vi "Просмотр графиков2.vi"(7 "tdm":string) -> ()   [LabVIEW 2011]
panel:
  out "т1 2":waveform(dbl)[](graph)
  out "т1":waveform(dbl)[](graph)
  in  "Закрыть окно":bool
  in  "Сохранить":bool
  # "С1"
  # "С2"
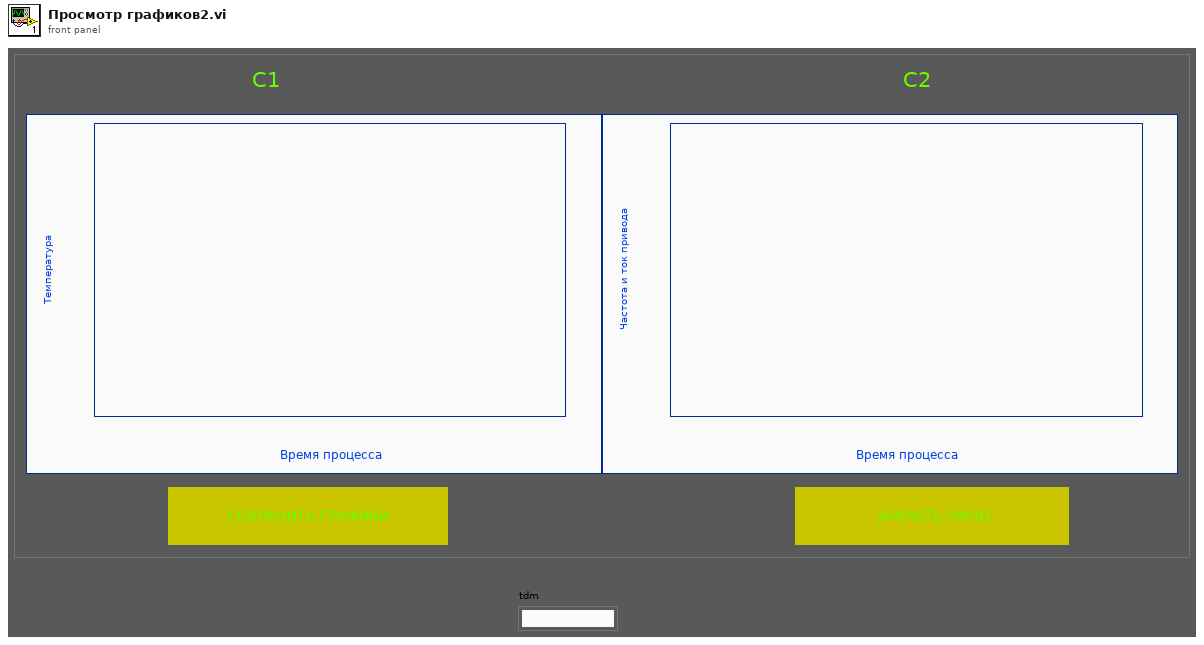
[diagram p1: front panel]
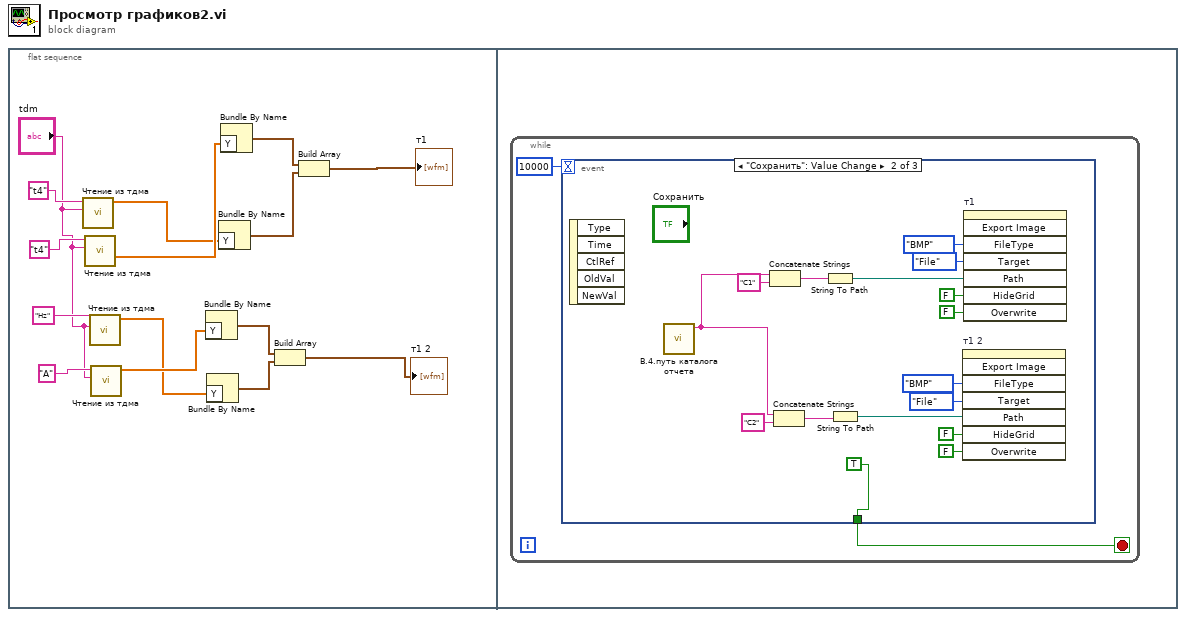
[diagram p0: block diagram]
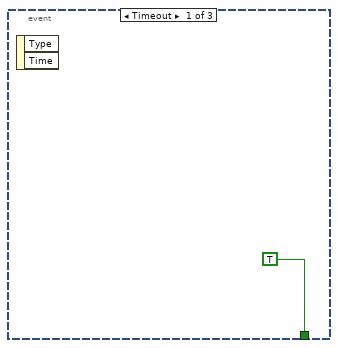
[diagram p2: hidden frame]
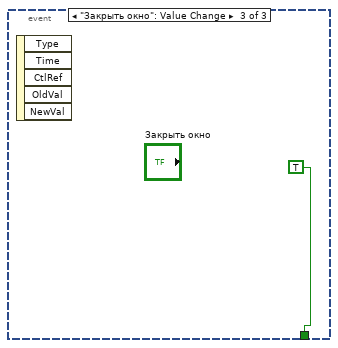
[diagram p3: hidden frame]
diagram:
  n1 = flat-sequence {
    frame #0 {
      n2 = call "Чтение из тдма.vi"("tdm"="tdm", "Канал"="t4") -> ("data"=w2:dbl[])  [unwired: 9 in]
      n3 = call "Чтение из тдма.vi"("tdm"="tdm", "Канал"="t4") -> ("data"=w3:dbl[])  [unwired: 9 in]
      n4 = call "Чтение из тдма.vi"("tdm"="tdm", "Канал"="Hz") -> ("data"=w4:dbl[])  [unwired: 9 in]
      n5 = call "Чтение из тдма.vi"("tdm"="tdm", "Канал"="A") -> ("data"=w5:dbl[])  [unwired: 9 in]
      n6 = Bundle By Name("Y"=w5) -> (w7:waveform(dbl))  [unwired: 1 in]
      n7 = Bundle By Name("Y"=w4) -> (w8:waveform(dbl))  [unwired: 1 in]
      n8 = Bundle By Name("Y"=w2) -> (w12:waveform(dbl))  [unwired: 1 in]
      n9 = Bundle By Name("Y"=w3) -> (w13:waveform(dbl))  [unwired: 1 in]
      n10 = Build Array(w7, w8) -> (→"т1 2":waveform(dbl)[])
      n11 = Build Array(w13, w12) -> (→"т1":waveform(dbl)[])
    }
    frame #1 {
      n12 = while {
        stop <- w16 stop-if-true
        n13 = event shown="[1] \"Сохранить\": Value Change" {
          selector: _ -> [_ _ _]
          dyn-events: _ -> [_ _ _]
          timeout: 10000 -> [_ _ _]
          tunnel: [TRUE TRUE TRUE] -> w16
          event Timeout {
            n14 = event-data() -> ()  [unwired: 1 in, 2 out]
          }
          event "Сохранить": Value Change {
            n15 = event-data() -> ()  [unwired: 1 in, 5 out]
            n16 = call "B.4.путь каталога отчета.vi"() -> ("path_out"=w22:string)  [unwired: 11 in]
            n17 = Concatenate Strings(w22, "C1" ("string")) -> (w24:string)
            n18 = Concatenate Strings(w22, "C2" ("string")) -> (w26:string)
            n19 = String To Path(string=w24) -> (path=w23:path)
            n20 = String To Path(string=w26) -> (path=w25:path)
            n21 = invoke on="т1 2" class="WFGraph (strict)" method="Export Image"("FileType"=enum32{"BMP", "EPS", "EMF", "PICT"}."BMP" ("File Type"), "Target"=enum32{"File", "Clipboard"}."File", "Path"=w25, "HideGrid"=FALSE ("Hide Grid"), "Overwrite"=FALSE ("Always Overwrite")) -> ()  [unwired: 3 in, 8 out]
            n22 = invoke on="т1" class="WFGraph (strict)" method="Export Image"("FileType"=enum32{"BMP", "EPS", "EMF", "PICT"}."BMP" ("File Type"), "Target"=enum32{"File", "Clipboard"}."File", "Path"=w23, "HideGrid"=FALSE ("Hide Grid"), "Overwrite"=FALSE ("Always Overwrite")) -> ()  [unwired: 3 in, 8 out]
          }
          event "Закрыть окно": Value Change {
            n23 = event-data() -> ()  [unwired: 1 in, 5 out]
          }
        }
      }
    }
  }
